vi "Stop Core.vi"(10 "final error code":i32, 11 "Actor in":refnum<class "RefNums and UICtrl.lvclass">) -> (3 "Actor out":refnum<class "RefNums and UICtrl.lvclass">)   [LabVIEW 2020, in "RefNums and UICtrl.lvclass"]
doc: "(<B>Filename</B>: Actor Framework.lvlib:Actor.lvclass:Stop Core.vi)\n\nDefines what the actor does before it stops. Use the <B>final error code</B> input to determine whether the actor shut down in response to an error.\n\nBy default, this method does nothing. A descendant class may override it to define behavior, such as shutting down any processes the actor initiated in its override of the Actor Core method."
uses:
  RefNums and UICtrl.lvclass
  <vilib>/MGI/Monitored Actor/Monitored Actor/Monitored Actor/Monitored Actor.lvclass
  RefNums and UICtrl.lvclass/RefNums and UICtrl.ctl
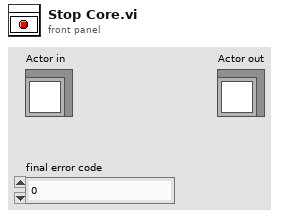
[diagram p1: front panel]
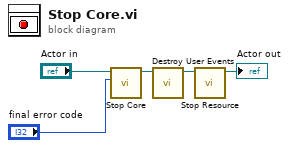
[diagram p0: block diagram]
diagram:
  n1 = call-parent "Stop Core.vi"("final error code"="final error code", "Monitored Actor in"="Actor in") -> ("Monitored Actor out"=w3:refnum<class "RefNums and UICtrl.lvclass">)  [unwired: 9 in]
  n2 = call "Destroy User Events.vi"("Actor in"=w3) -> ("Actor out"=w2:refnum<class "RefNums and UICtrl.lvclass">)  [unwired: 10 in]
  n3 = call "Stop Resource.vi"("Actor in"=w2) -> ("Actor out"=→"Actor out":refnum<class "RefNums and UICtrl.lvclass">)  [unwired: 10 in]
